vi "XNET Frame to Signal.vi"(8 "error in (no error)":errorcluster, 10 "Frame":string, 11 "CAN in":refnum<class "XNET_BS120x.lvclass">) -> (0 "error out":errorcluster, 2 "signal data":dbl[](array[numeric]), 3 "CAN out":refnum<class "XNET_BS120x.lvclass">)   [LabVIEW 2021, in "BS120x Driver.lvlib" / "XNET_BS120x.lvclass"]
uses:
  XNET_BS120x.lvclass
  XNET_BS120x.lvclass/XNET_BS120x.ctl
  _Private/Data Classes/XNET Data Class/XNET Data.lvclass/XNET Data.ctl
  _Private/Data Classes/XNET Data Class/Read XNET Array.vi
  <vilib>/xnet/xnet.llb/XNET Create Session (Conversion).vi
  <vilib>/xnet/xnet.llb/XNET Convert (Frame CAN to Signal).vi
  _Private/Data Classes/XNET Data Class/XNET Data.lvclass
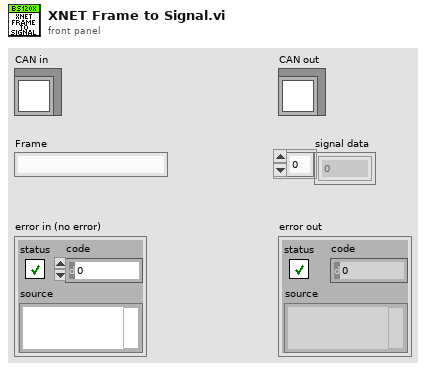
[diagram p1: front panel]
types:
  T1 = typedef "XNET Frame CAN.ctl" = cluster{"timestamp":timestamp, "payload":u8[], "identifier":u32, "type":T2, "extended?":bool, "echo?":bool}
  T2 = typedef "XNET Frame Type CAN.ctl" = u8
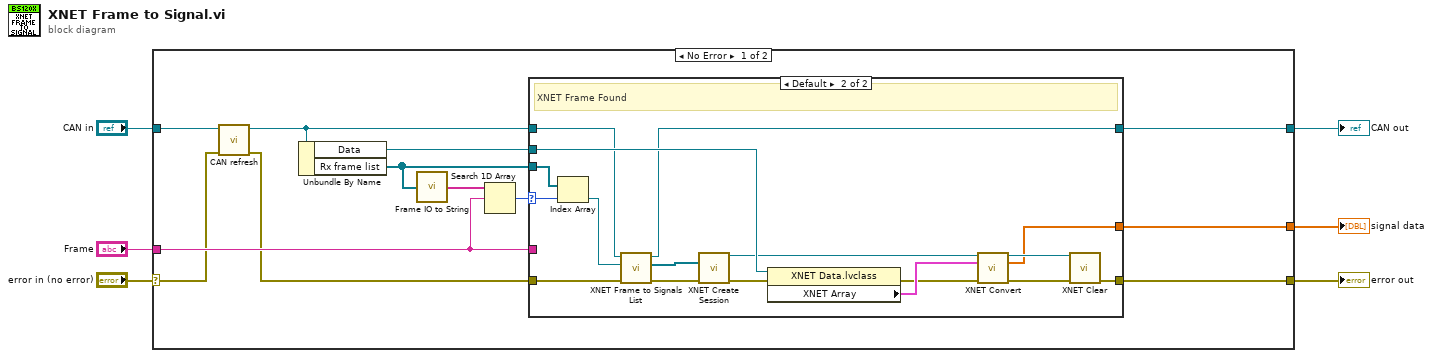
[diagram p0: block diagram]
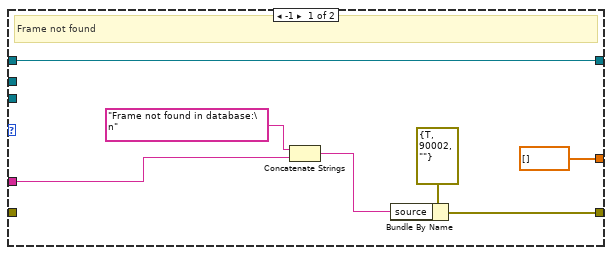
[diagram p2: hidden frame]
diagram:
  n1 = case shown="No Error" "error in (no error)" {
    selector: "error in (no error)" -> [w8 w44]
    tunnel: [w12 w44] -> w4
    tunnel: [w11 w43] -> w1
    tunnel: "CAN in" -> [w10 w43]
    tunnel: "Frame" -> [w16 _]
    tunnel: [w18 _] -> w3
    frame No Error {
      n2 = call "CAN refresh.vi"("error in (no error)"=w8, "CAN in"=w10) -> ("error out"=w7:errorcluster, "CAN out"=w9:refnum<class "XNET_BS120x.lvclass">)  [unwired: 8 in]
      n3 = Unbundle By Name(w9) -> ("Data"=w13:refnum<class "XNET Data.lvclass">, "Rx frame list"=w17:refnum<k21>[])
      n4 = call "Frame IO to String.vi"("Frame list"=w17) -> ("Frame list"=w14:string[])
      n5 = Search 1D Array(1D array=w14, element=w16) -> (index of element=w15:i32)  [unwired: 1 in]
      n6 = case shown="Default" w15 {
        selector: w15 -> [_ w35]
        tunnel: [dbl[] [] ("signal data") w41] -> w18
        tunnel: w13 -> [_ w33]
        tunnel: [w21 w37] -> w12
        tunnel: w17 -> [_ w36]
        tunnel: w16 -> [w20 _]
        tunnel: w7 -> [_ w34]
        tunnel: w9 -> [w19 w28]
        tunnel: [w19 w27] -> w11
        frame -1 {
          # "Frame not found"
          n7 = Concatenate Strings("Frame not found in database:\n" ("source"), w20) -> (w22:string)
          n8 = Bundle By Name(cluster=errorcluster {"status"=TRUE, "code"=90002, "source"=""} ("error out"), "source"=w22) -> (w21:errorcluster)
        }
        frame Default {
          # "XNET Frame Found"
          n9 = Index Array(array=w36, index=w35) -> (element=w29:refnum<k21>)
          n10 = call-dynamic "XNET Frame to Signals List.vi"("error in (no error)"=w34, "XNET Frame"=w29, "BS1200 in"=w28) -> ("error out"=w39:errorcluster, "Sorted XNET Signals"=w26:refnum<k21>[], "BS1200 out"=w27:refnum<class "XNET_BS120x.lvclass">)  [unwired: 6 in]
          n11 = call-poly <vilib>:"XNET Create Session.vi"("signal list"=w26, "error in (no error)"=w39) -> ("session out"=w32:refnum<k21>, "error out"=w31:errorcluster)  [unwired: 12 out]
          n12 = property class="XNET Data.lvclass"(reference=w33, error in=w31) -> (error out=w30:errorcluster, "XNET Array"=w40:T1[])  [unwired: 1 out]
          n13 = call-poly <vilib>:"XNET Convert.vi"("session in"=w32, "frame data"=w40, "error in (no error)"=w30) -> ("session out"=w42:refnum<k21>, "signal data"=w41:dbl[], "error out"=w38:errorcluster)  [unwired: 10 out]
          n14 = call <vilib>:"XNET Clear.vi"("session in"=w42, "error in (no error)"=w38) -> ("error out"=w37:errorcluster)  [unwired: 13 in]
        }
      }
    }
    frame Error {
    }
  }
  "error out" <- w4
  "signal data" <- w3
  "CAN out" <- w1
